vi "GLdrv_SCAL_FUNC.vi"(0 "Connection ID":T1, 5 "CH":i32=1 min=1, 7 "Function":enum16{"ON", "OFF"}(ring), 11 "error in (no error)":errorcluster, 13 "Query(f)":bool) -> (4 "Connection ID Out":T1, 8 "Function out":enum16{"ON", "OFF"}(ring), 15 "error out":errorcluster)   [LabVIEW 2017, in "GL860_Driver.lvlib"]
doc: "スケーリングのOn/Offの設定・参照\nOff/ON\n例）　:SCAL:CH1:FUNC ON (アナログ入力CH1のスケーリング機\n能をONにします)"
uses:
  GL860_Driver.lvlib
  ConnectionID.ctl
  GLdrv_RW.ctl
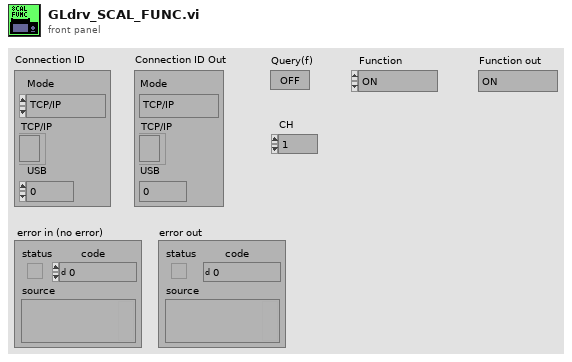
[diagram p1: front panel]
types:
  T1 = typedef "ConnectionID.ctl" = cluster{"Mode":enum16{"TCP/IP", "USB"}, "TCP/IP":refnum<k5>, "USB":i32}
  T2 = typedef "GLdrv_RW.ctl" = enum16{"Auto", "Read", "Write", "Buffer"}
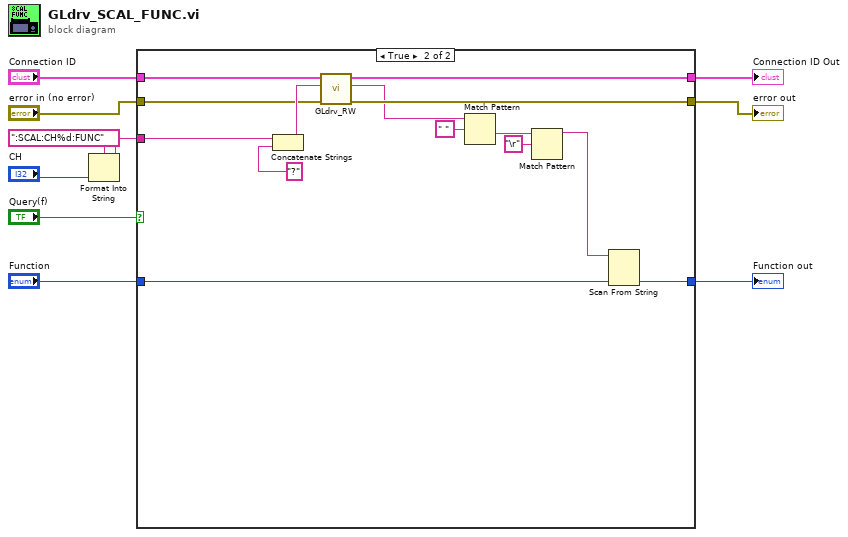
[diagram p0: block diagram]
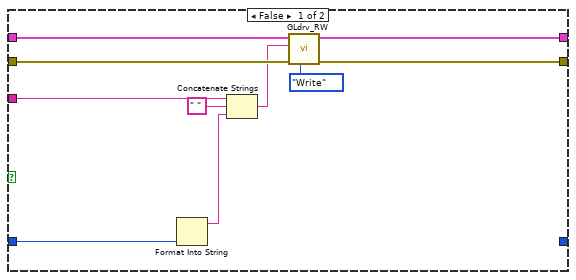
[diagram p2: hidden frame]
diagram:
  n1 = Format Into String(format string=":SCAL:CH%d:FUNC" ("Command"), "CH") -> (resulting string=w5:string)  [unwired: 2 in, 1 out]
  n2 = case shown="TRUE" "Query(f)" {
    tunnel: w5 -> [w20 w34]
    tunnel: [w15 w28] -> w10
    tunnel: [w17 w31] -> w9
    tunnel: "Connection ID" -> [w18 w32]
    tunnel: "error in (no error)" -> [w16 w29]
    tunnel: "Function" -> [w11 w27]
    tunnel: [_ w26] -> w2
    frame False {
      n3 = Format Into String(w11) -> (resulting string=w12:string)  [unwired: 3 in, 1 out]
      n4 = Concatenate Strings(w20, " " ("string"), w12) -> (w14:string)
      n5 = call "GLdrv_RW.vi"("Mode(read)"=GLdrv_RW."Write", "error in (no error)"=w16, "data in"=w14, "Connection ID"=w18) -> ("error out"=w15:errorcluster, "Connection ID Out"=w17:T1)  [unwired: 3 in, 3 out]
    }
    frame True {
      n6 = Concatenate Strings(w34, "?" ("string")) -> (w30:string)
      n7 = call "GLdrv_RW.vi"("error in (no error)"=w29, "data in"=w30, "Connection ID"=w32) -> ("error out"=w28:errorcluster, "data out"=w21:string, "Connection ID Out"=w31:T1)  [unwired: 4 in, 2 out]
      n8 = Match Pattern(string=w21, regular expression=" " ("search string/char (-)")) -> (after substring=w23:string)  [unwired: 4 out]
      n9 = Match Pattern(string=w23, regular expression="\r") -> (before substring=w22:string)  [unwired: 4 out]
      n10 = Scan From String(input string=w22, default 1=w27) -> (output 1=w26:enum16{"ON", "OFF"})  [unwired: 3 in, 3 out]
    }
  }
  "Connection ID Out" <- w9
  "error out" <- w10
  "Function out" <- w2
